vi "Continuous.vi"(8 "error in (no error)":errorcluster, 10 "Power Supply in":refnum<class "Power Supply.lvclass">, 11 "Continuous.lvclass in":refnum<class "Magnetic Field Oxford Continuous.lvclass">) -> (0 "error out":errorcluster, 3 "Continuous.lvclass out":refnum<class "Magnetic Field Oxford Continuous.lvclass">)   [LabVIEW 2023, in "Magnetic Field Oxford Continuous.lvclass"]
uses:
  Magnetic Field Oxford Continuous.lvclass
  C:/LabVIEW-programs/Scanners/Scanner/Scanner.lvclass
  Instruments/Oxford Magnet/Power Supply/Power Supply.lvclass
  C:/LabVIEW-programs/Instruments/Utility Classes/Scannable/Scannable.lvclass
  Scanner/Scanner.lvclass
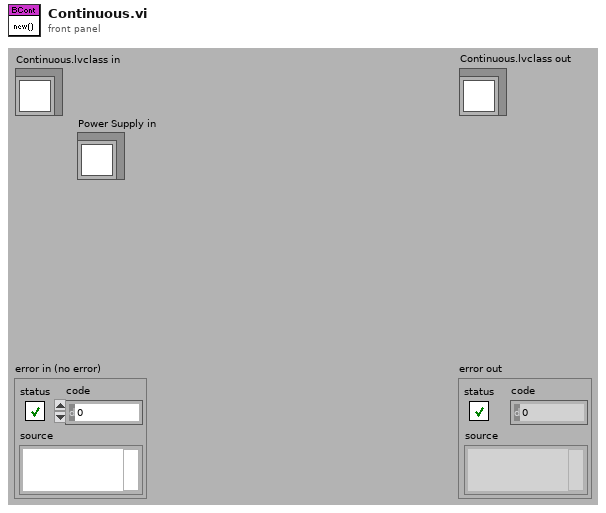
[diagram p1: front panel]
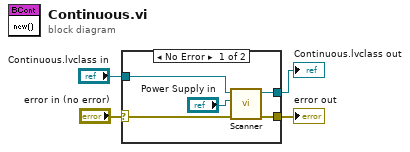
[diagram p0: block diagram]
diagram:
  n1 = case shown="No Error" "error in (no error)" {
    selector: "error in (no error)" -> [w7 w10]
    tunnel: [w6 w10] -> w3
    tunnel: [w8 w11] -> w1
    tunnel: "Continuous.lvclass in" -> [w9 w11]
    frame No Error {
      n2 = call "Scanner.vi"("error in (no error)"=w7, "Scannable"="Power Supply in", "Scanner.lvclass in"=w9) -> ("error out"=w6:errorcluster, "Scanner.lvclass out"=w8:refnum<class "Magnetic Field Oxford Continuous.lvclass">)  [unwired: 1 in, 6 out]
    }
    frame Error {
    }
  }
  "error out" <- w3
  "Continuous.lvclass out" <- w1
